vi "Event Generate.vi"(9 "Msg":refnum<class "Msg.lvclass">, 10 "Event":refnum<data-value>) -> (0 "error out":errorcluster)   [LabVIEW 2021, in "jettl.lvlib"]
uses:
  jettl.lvlib
  Msg/Msg/Msg.lvclass
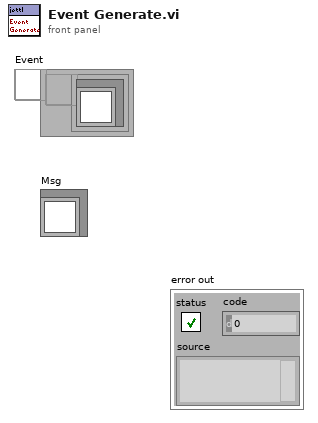
[diagram p1: front panel]
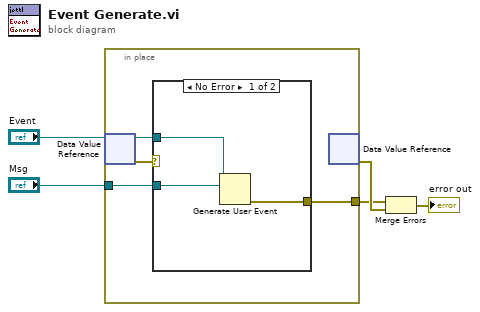
[diagram p0: block diagram]
diagram:
  n1 = in-place {
    in-place-border: "Msg" -> [w9]
    in-place-border: [w8] -> w3
    n2 = in-place-dvr #1("Event") -> (w7:refnum<user-event>, w6:errorcluster)
    n3 = case shown="No Error" w6 {
      selector: w6 -> [_ w13]
      tunnel: w9 -> [w12 _]
      tunnel: [w11 w13] -> w8
      tunnel: w7 -> [w10 _]
      frame No Error {
        n4 = Generate User Event(user event=w10, event data cluster=w12) -> (error out=w11:errorcluster)  [unwired: 2 in, 1 out]
      }
      frame Error {
      }
    }
    n5 = in-place-dvr #1() -> (w4:errorcluster)  [unwired: 1 in, 1 out]
  }
  n6 = Merge Errors(w3, w4) -> (→"error out":errorcluster)
